vi "Force sensing Resistor FPGA.vi"() -> ()   [LabVIEW 2018, in "jmslib.lvlib"]
uses:
  jmslib.lvlib
  <vilib>/rvi/eio/common/nirviEmuTemplateMethod_errors.vi
  <vilib>/eio/EIONode/EIONode.xnode
panel:
  out "I/O Item":i16
  in  "FPGA I/O In":refnum<k21>="Connector0/AI0"
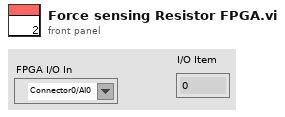
[diagram p1: front panel]
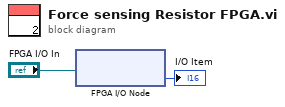
[diagram p0: block diagram]
diagram:
  n1 = xnode "FPGA I/O Node"("FPGA I/O In"="FPGA I/O In") -> ("I/O Item"=→"I/O Item":i16)  [unwired: 1 out]
